vi "Update Service Info.vi"(8 "error in (no error)":errorcluster, 9 "Port":i32, 10 "Type":T1, 11 "DiscoveryService in":refnum<class "DiscoveryService.lvclass">) -> (0 "error out":errorcluster, 3 "DiscoveryService out":refnum<class "DiscoveryService.lvclass">)   [LabVIEW 2020, in "Vecto.lvlib" / "DiscoveryService.lvclass"]
uses:
  DiscoveryService.lvclass
  proto/ServiceType/Enumeration.ctl
  Update Service Data.ctl
  proto/Service/Data.ctl
  DiscoveryService.lvclass/DiscoveryService.ctl
  proto/ServiceType/ServiceType.lvlib
  proto/Service/Service.lvlib
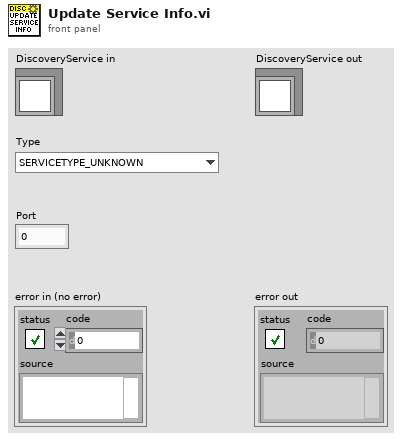
[diagram p1: front panel]
types:
  T1 = typedef "ServiceType.lvlib/Enumeration.ctl" = enum16{"SERVICETYPE_UNKNOWN", "SERVICETYPE_TCPSERVER", "SERVICETYPE_HTTPSERVER"}
  T2 = typedef "Vecto.lvlib/DiscoveryService.lvclass/Update Service Data.ctl" = cluster{"Service":T3}
  T3 = typedef "Service.lvlib/Data.ctl" = cluster{"type":T1, "port":i32}
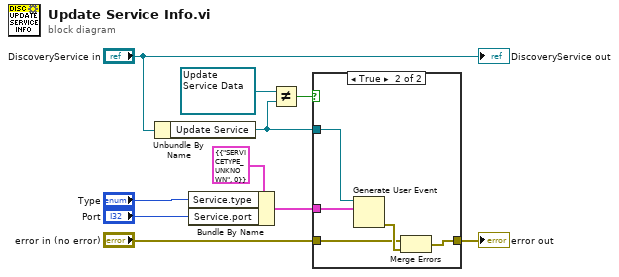
[diagram p0: block diagram]
diagram:
  n1 = Unbundle By Name("DiscoveryService in") -> ("Update Service"=w3:refnum<user-event>)
  n2 = Bundle By Name(cluster=T2 {"Service"={"type"=enum."SERVICETYPE_UNKNOWN", "port"=0}} ("event data"), "Service.type"="Type", "Service.port"="Port") -> (w9:T2)
  n3 = Not Equal?(x=refnum<user-event> refnum, y=w3) -> (x != y?=w1:bool)
  n4 = case shown="True" w1 {
    tunnel: w9 -> [_ w16]
    tunnel: "error in (no error)" -> [w11 w14]
    tunnel: [w11 w13] -> w7
    tunnel: w3 -> [_ w12]
    frame False {
    }
    frame True {
      n5 = Generate User Event(user event=w12, event data cluster=w16) -> (error out=w15:errorcluster)  [unwired: 2 in, 1 out]
      n6 = Merge Errors(w14, w15) -> (w13:errorcluster)
    }
  }
  "error out" <- w7
  "DiscoveryService out" <- "DiscoveryService in"
